vi "SortToneDataForLogging.vi"(7 "Target":T1=enum."4", 10 "element in":cluster{"Enum":T5, "Data":variant}, 11 "TonesLog":T2={"72co"={"Count"=0, "CalVal"=[], "CalLoc"=[], "BeacVal"=[], "BeacLoc"=[], "BeacShift"=[], "Enum"=enum."4", "df"=0.0, "PwrSpectr"=[], "ISpectr"=[], "QSpectr"=[], "Time"=[], "SNR"=[], "AboveThresh"=[], "10Hz_PeakVal"=[], "Phase"=[], "DeltaPhase"=[], "Saturat"={"Meas"=[], "Stage1"=[], "Stage4"=[], "Stage5"=[], "Stage6"=[], "Stage7"=[]}, "10MHz"=FALSE}, "72x"={"Count"=0, "CalVal"=[], "CalLoc"=[], "BeacVal"=[], "BeacLoc"=[], "BeacShift"=[], "Enum"=enum."4", "df"=0.0, "PwrSpectr"=[], "ISpectr"=[], "QSpectr"=[], "Time"=[], "SNR"=[], "AboveThresh"=[], "10Hz_PeakVal"=[], "Phase"=[], "DeltaPhase"=[], "Saturat"={"Meas"=[], "Stage1"=[], "Stage4"=[], "Stage5"=[], "Stage6"=[], "Stage7"=[]}, "10MHz"=FALSE}, "84co"={"Count"=0, "CalVal"=[], "CalLoc"=[], "BeacVal"=[], "BeacLoc"=[], "BeacShift"=[], "Enum"=enum."4", "df"=0.0, "PwrSpectr"=[], "ISpectr"=[], "QSpectr"=[], "Time"=[], "SNR"=[], "AboveThresh"=[], "10Hz_PeakVal"=[], "Phase"=[], "DeltaPhase"=[], "Saturat"={"Meas"=[], "Stage1"=[], "Stage4"=[], "Stage5"=[], "Stage6"=[], "Stage7"=[]}, "10MHz"=FALSE}, "84x"={"Count"=0, "CalVal"=[], "CalLoc"=[], "BeacVal"=[], "BeacLoc"=[], "BeacShift"=[], "Enum"=enum."4", "df"=0.0, "PwrSpectr"=[], "ISpectr"=[], "QSpectr"=[], "Time"=[], "SNR"=[], "AboveThresh"=[], "10Hz_PeakVal"=[], "Phase"=[], "DeltaPhase"=[], "Saturat"={"Meas"=[], "Stage1"=[], "Stage4"=[], "Stage5"=[], "Stage6"=[], "Stage7"=[]}, "10MHz"=FALSE}}) -> (1 "SendToQueue":cluster{"Enum":T5, "Data":variant}, 2 "Full set":bool, 3 "TonesLog w/ New Data":T2={"72co"={"Count"=0, "CalVal"=[], "CalLoc"=[], "BeacVal"=[], "BeacLoc"=[], "BeacShift"=[], "Enum"=enum."4", "df"=0.0, "PwrSpectr"=[], "ISpectr"=[], "QSpectr"=[], "Time"=[], "SNR"=[], "AboveThresh"=[], "10Hz_PeakVal"=[], "Phase"=[], "DeltaPhase"=[], "Saturat"={"Meas"=[], "Stage1"=[], "Stage4"=[], "Stage5"=[], "Stage6"=[], "Stage7"=[]}, "10MHz"=FALSE}, "72x"={"Count"=0, "CalVal"=[], "CalLoc"=[], "BeacVal"=[], "BeacLoc"=[], "BeacShift"=[], "Enum"=enum."4", "df"=0.0, "PwrSpectr"=[], "ISpectr"=[], "QSpectr"=[], "Time"=[], "SNR"=[], "AboveThresh"=[], "10Hz_PeakVal"=[], "Phase"=[], "DeltaPhase"=[], "Saturat"={"Meas"=[], "Stage1"=[], "Stage4"=[], "Stage5"=[], "Stage6"=[], "Stage7"=[]}, "10MHz"=FALSE}, "84co"={"Count"=0, "CalVal"=[], "CalLoc"=[], "BeacVal"=[], "BeacLoc"=[], "BeacShift"=[], "Enum"=enum."4", "df"=0.0, "PwrSpectr"=[], "ISpectr"=[], "QSpectr"=[], "Time"=[], "SNR"=[], "AboveThresh"=[], "10Hz_PeakVal"=[], "Phase"=[], "DeltaPhase"=[], "Saturat"={"Meas"=[], "Stage1"=[], "Stage4"=[], "Stage5"=[], "Stage6"=[], "Stage7"=[]}, "10MHz"=FALSE}, "84x"={"Count"=0, "CalVal"=[], "CalLoc"=[], "BeacVal"=[], "BeacLoc"=[], "BeacShift"=[], "Enum"=enum."4", "df"=0.0, "PwrSpectr"=[], "ISpectr"=[], "QSpectr"=[], "Time"=[], "SNR"=[], "AboveThresh"=[], "10Hz_PeakVal"=[], "Phase"=[], "DeltaPhase"=[], "Saturat"={"Meas"=[], "Stage1"=[], "Stage4"=[], "Stage5"=[], "Stage6"=[], "Stage7"=[]}, "10MHz"=FALSE}}, 4 "Target":T1=enum."4", 5 "10Hz_Time":timestamp, 6 "10Hz_PeakVal":dbl[](array[numeric]))   [LabVIEW 2018]
uses:
  Controls/Enums/LogLoopEnum.ctl
  Controls/Clusts/TonesLogAll.ctl
  Controls/Clusts/ToneLogBuffered.ctl
  Controls/Enums/TargetNumber.ctl
  Controls/Clusts/SaturationMonitorBuffer.ctl
  Controls/Clusts/TargetToneData.ctl
  Controls/Clusts/ChannelToneData.ctl
  Controls/ToneInfoClust.ctl
  Controls/Clusts/SaturationMonitor.ctl
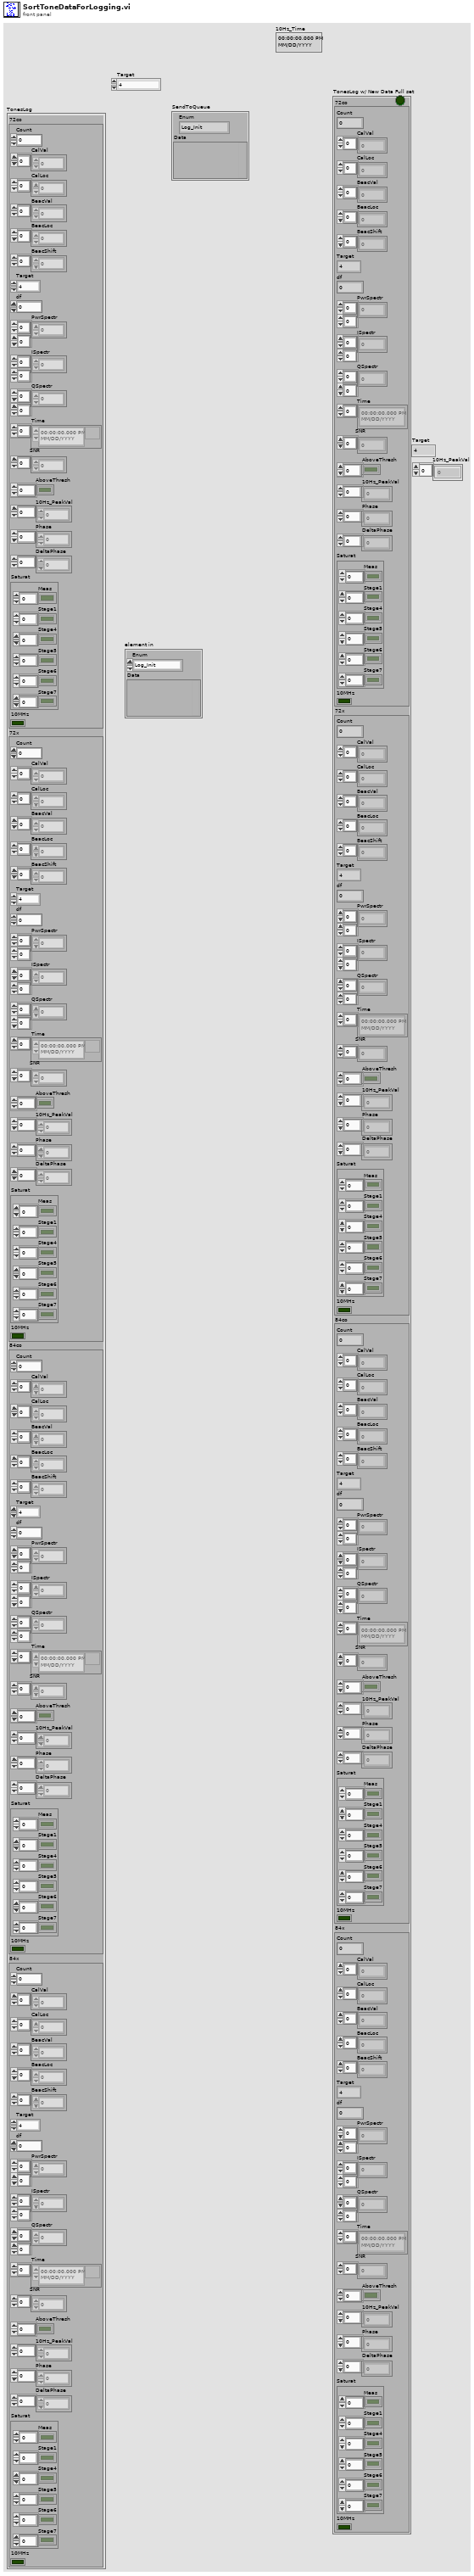
[diagram p1: front panel]
types:
  T1 = typedef "TargetNumber.ctl" = enum16{"1", "2", "3", "4"}
  T2 = typedef "TonesLogAll.ctl" = cluster{"72co":T3, "72x":T3, "84co":T3, "84x":T3}
  T3 = typedef "ToneLogBuffered.ctl" = cluster{"Count":i32, "CalVal":sgl[], "CalLoc":i32[], "BeacVal":sgl[], "BeacLoc":i32[], "BeacShift":i32[], "Enum":T1, "df":dbl, "PwrSpectr":sgl[][], "ISpectr":sgl[][], "QSpectr":sgl[][], "Time":timestamp[], "SNR":sgl[], "AboveThresh":bool[], "10Hz_PeakVal":dbl[], "Phase":sgl[], "DeltaPhase":dbl[], "Saturat":T4, "10MHz":bool}
  T4 = typedef "SaturationMonitorBuffer.ctl" = cluster{"Meas":bool[], "Stage1":bool[], "Stage4":bool[], "Stage5":bool[], "Stage6":bool[], "Stage7":bool[]}
  T5 = typedef "LogLoopEnum.ctl" = enum16{"Log_Init", "Log_Config", "Log_CfgAlarm", "Log_TimeDomain", "Log_Tone", "Log_NoiseTrace", "Log_NoiseSum", "Log_DO", "Log_AI", "Log_TC", "Log_Disdrom", "Log_Weather", "Log_TE", "Log_ADAM", "Log_UPS", "Log_ChkTime", "Log_Alarm", "Log_SSH", "Log_Write", "Log_Exit"}
  T6 = typedef "TargetToneData.ctl" = cluster{"Cal":T7, "Beac":T7, "Time":timestamp[], "Saturat":T9}
  T7 = typedef "ChannelToneData.ctl" = cluster{"Shift_":dbl, "Peak_ToFPGA":dbl, "MaxValue":dbl, "MaxIndex":i32, "Tone":T8, "TimeDomainI":ext[], "TimeDomainQ":ext[], "PwrSpectrum":dbl[], "RunningAvgFreq":dbl, "ISpectPos":dbl[], "ISpectNeg":dbl[], "QSpectPos":dbl[], "QSpectNeg":dbl[], "10Hz_PwrSpectr":dbl[][], "SNR":dbl, "AliasWarn":bool, "10Hz_Peak":dbl[], "ISpect+-":dbl[], "QSpect+-":dbl[], "TimeStamp":timestamp, "I_Index":ext[], "Q_Index":ext[], "10MHz":bool}
  T8 = typedef "ToneInfoClust.ctl" = cluster{"PkLocTrak":dbl, "PkLocDisp":dbl, "df_":dbl, "ZoomPwr":dbl[], "Phase":dbl, "PhaseOld":dbl, "AboveThresh?":bool, "MaxI":dbl, "MaxQ":dbl, "median":dbl, "ISpect":dbl[], "QSpect":dbl[], "DeltaPhase":dbl}
  T9 = typedef "SaturationMonitor.ctl" = cluster{"MeasMean0":dbl, "MeasMean1":dbl, "MeasMax":dbl, "1_Max":dbl, "4_Max":dbl, "5_Max":dbl, "6_Max":dbl, "7_Max":dbl}
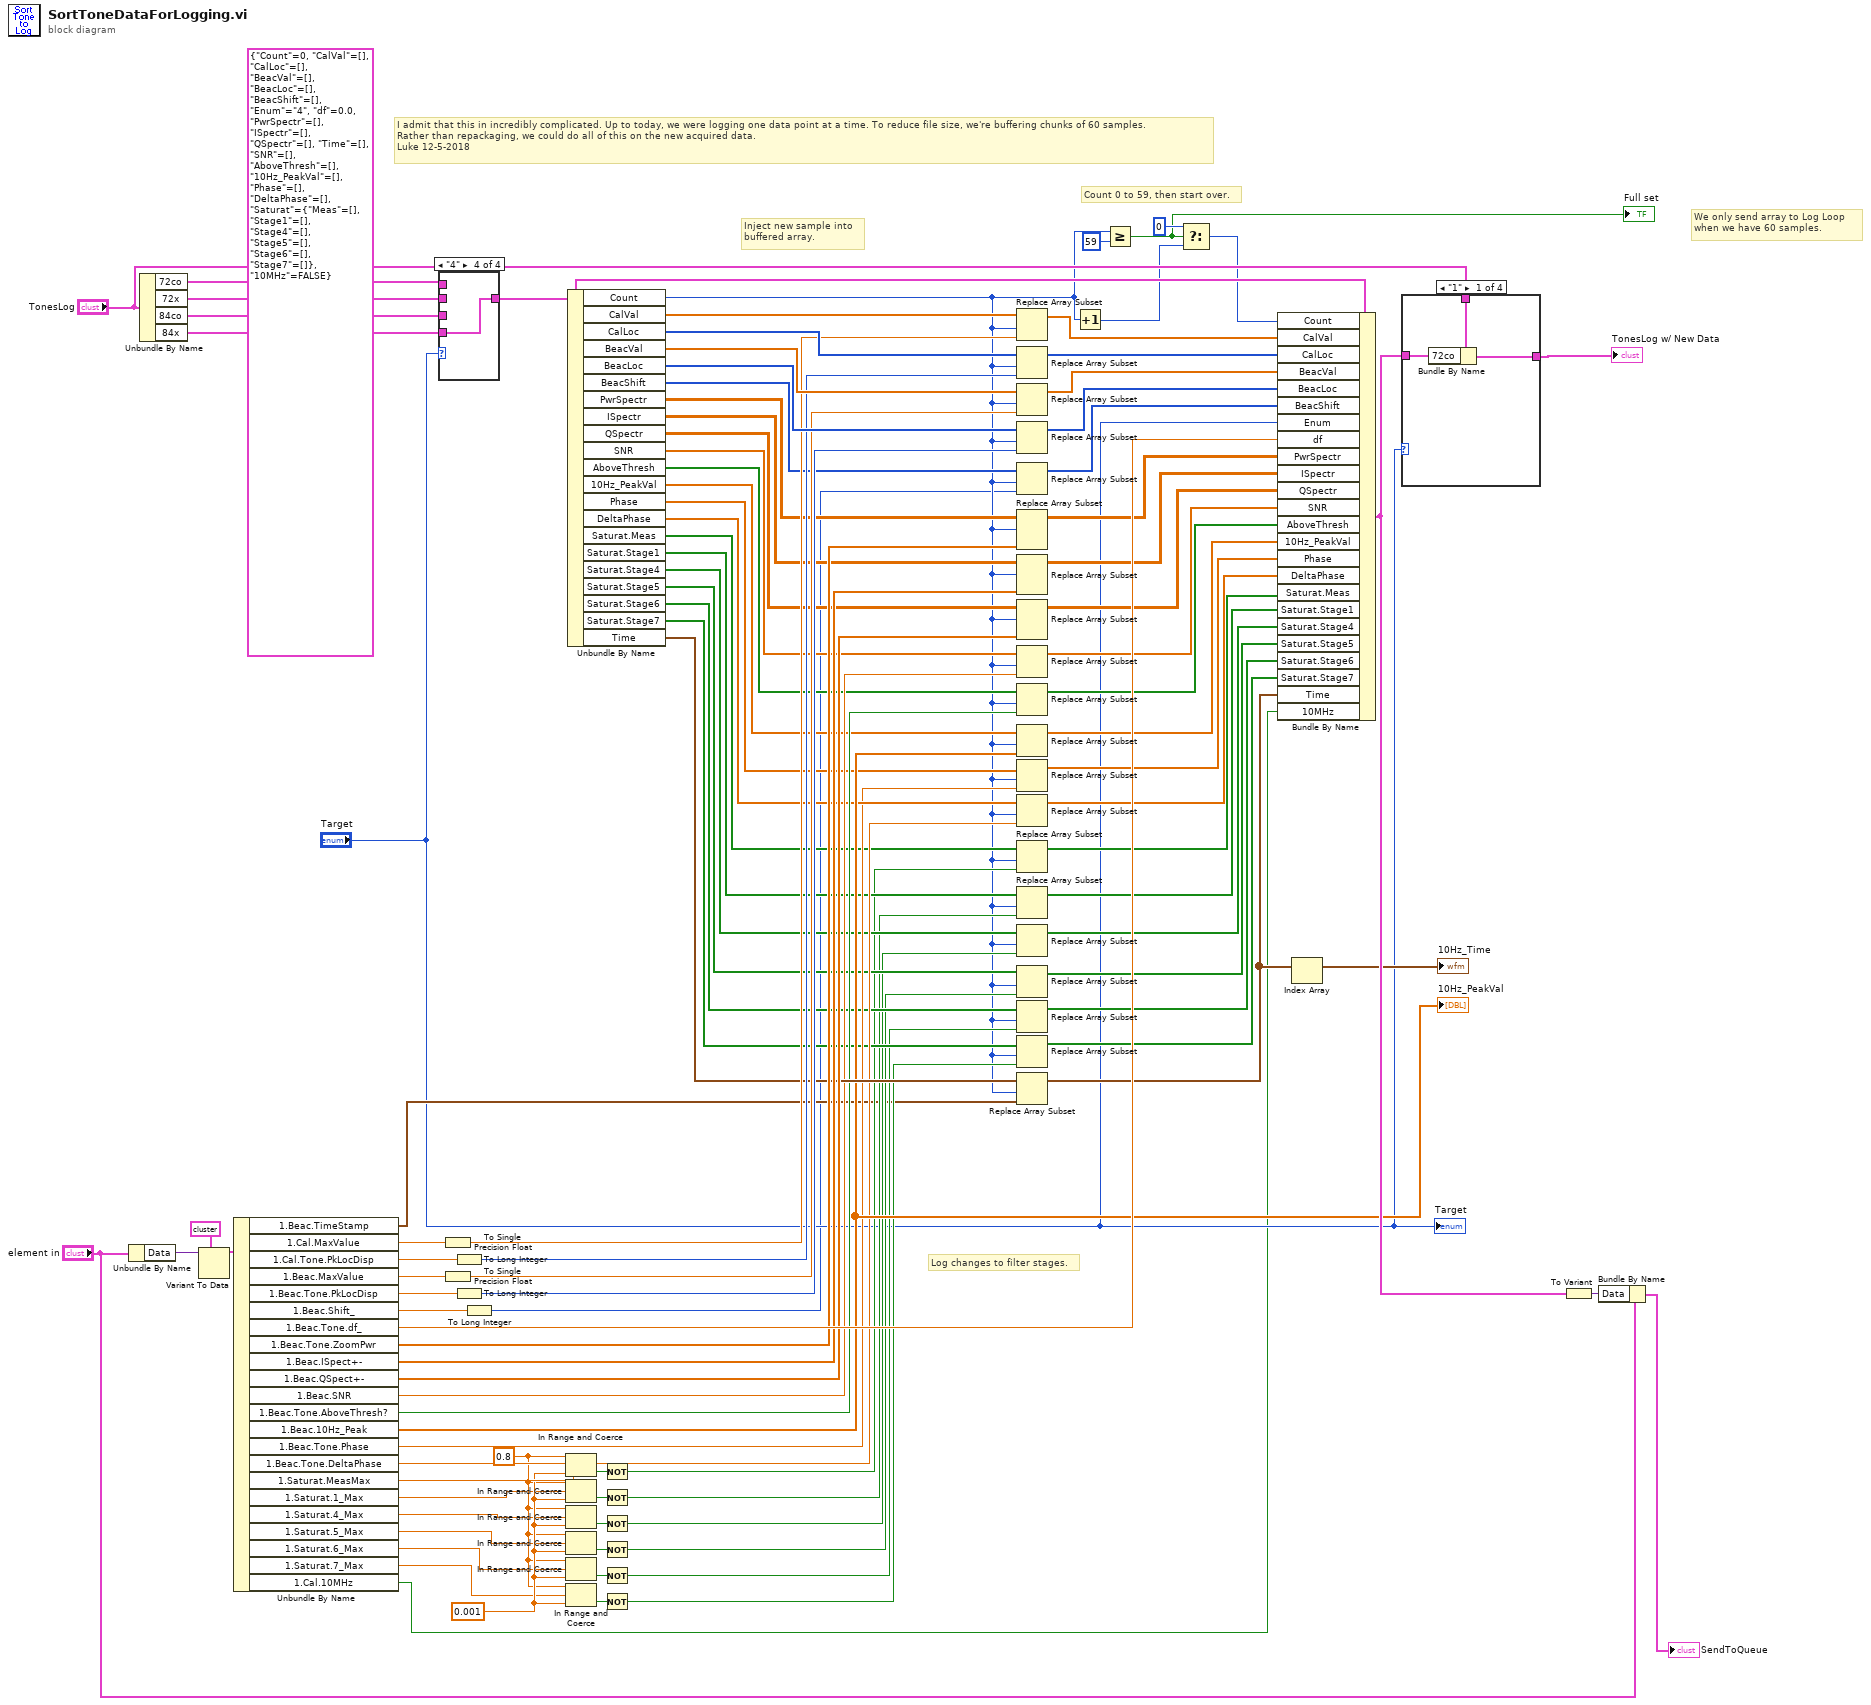
[diagram p0: block diagram]
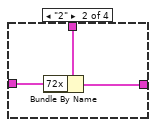
[diagram p2: hidden frame]
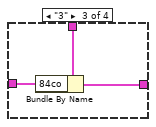
[diagram p3: hidden frame]
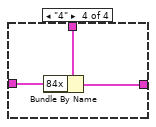
[diagram p4: hidden frame]
diagram:
  (unwired) T3 {"Count"=0, "CalVal"=[], "CalLoc"=[], "BeacVal"=[], "BeacLoc"=[], "BeacShift"=[], "Enum"=enum."4", "df"=0.0, "PwrSpectr"=[], "ISpectr"=[], "QSpectr"=[], "Time"=[], "SNR"=[], "AboveThresh"=[], "10Hz_PeakVal"=[], "Phase"=[], "DeltaPhase"=[], "Saturat"={"Meas"=[], "Stage1"=[], "Stage4"=[], "Stage5"=[], "Stage6"=[], "Stage7"=[]}, "10MHz"=FALSE} ("84x")
  w41 = 0.001 ("upper limit")
  w40 = 0.8 ("upper limit")
  # "Log changes to filter stages."
  # "We only send array to Log Loop\nwhen we have 60 samples."
  # "Inject new sample into\nbuffered array."
  # "Count 0 to 59, then start over."
  # "I admit that this in incredibly complicated. Up to today, we were logging one data point at a time. To reduce file size, we're buffering chunks of 60 samples.\nRather than repackaging, we could do all of this on the new acquired data.\nLuke 12-5-2018"
  n1 = Unbundle By Name("element in") -> ("Data"=w98:variant)
  n2 = Unbundle By Name("TonesLog") -> ("72co"=w102:T3, "72x"=w101:T3, "84co"=w100:T3, "84x"=w99:T3)
  n3 = Variant To Data(type=cluster{"Target":T1, "1":T6} {"Target"=enum."1", "1"={"Cal"={"Shift_"=0.0, "Peak_ToFPGA"=0.0, "MaxValue"=0.0, "MaxIndex"=0, "Tone"={"PkLocTrak"=0.0, "PkLocDisp"=0.0, "df_"=0.0, "ZoomPwr"=[], "Phase"=0.0, "PhaseOld"=0.0, "AboveThresh?"=FALSE, "MaxI"=0.0, "MaxQ"=0.0, "median"=0.0, "ISpect"=[], "QSpect"=[], "DeltaPhase"=0.0}, "TimeDomainI"=[], "TimeDomainQ"=[], "PwrSpectrum"=[], "RunningAvgFreq"=0.0, "ISpectPos"=[], "ISpectNeg"=[], "QSpectPos"=[], "QSpectNeg"=[], "10Hz_PwrSpectr"=[], "SNR"=0.0, "AliasWarn"=FALSE, "10Hz_Peak"=[], "ISpect+-"=[], "QSpect+-"=[], "TimeStamp"=timestamp(0 s since 1904-01-01), "I_Index"=array[12500 elements], "Q_Index"=array[12500 elements], "10MHz"=FALSE}, "Beac"={"Shift_"=0.0, "Peak_ToFPGA"=0.0, "MaxValue"=0.0, "MaxIndex"=0, "Tone"={"PkLocTrak"=0.0, "PkLocDisp"=0.0, "df_"=0.0, "ZoomPwr"=[], "Phase"=0.0, "PhaseOld"=0.0, "AboveThresh?"=FALSE, "MaxI"=0.0, "MaxQ"=0.0, "median"=0.0, "ISpect"=[], "QSpect"=[], "DeltaPhase"=0.0}, "TimeDomainI"=[], "TimeDomainQ"=[], "PwrSpectrum"=[], "RunningAvgFreq"=0.0, "ISpectPos"=[], "ISpectNeg"=[], "QSpectPos"=[], "QSpectNeg"=[], "10Hz_PwrSpectr"=[], "SNR"=0.0, "AliasWarn"=FALSE, "10Hz_Peak"=[], "ISpect+-"=[], "QSpect+-"=[], "TimeStamp"=timestamp(0 s since 1904-01-01), "I_Index"=array[12500 elements], "Q_Index"=array[12500 elements], "10MHz"=FALSE}, "Time"=[], "Saturat"={"MeasMean0"=0.0, "MeasMean1"=0.0, "MeasMax"=0.0, "1_Max"=0.0, "4_Max"=0.0, "5_Max"=0.0, "6_Max"=0.0, "7_Max"=0.0}}} ("Target# and Tone Data"), Variant=w98) -> (data=w97:cluster{"Target":T1, "1":T6})  [unwired: 1 in, 1 out]
  n4 = Unbundle By Name(w97) -> ("1.Beac.TimeStamp"=w5:timestamp, "1.Cal.MaxValue"=w95:dbl, "1.Cal.Tone.PkLocDisp"=w89:dbl, "1.Beac.MaxValue"=w70:dbl, "1.Beac.Tone.PkLocDisp"=w71:dbl, "1.Beac.Shift_"=w7:dbl, "1.Beac.Tone.df_"=w69:dbl, "1.Beac.Tone.ZoomPwr"=w68:dbl[], "1.Beac.ISpect+-"=w67:dbl[], "1.Beac.QSpect+-"=w66:dbl[], "1.Beac.SNR"=w56:dbl, "1.Beac.Tone.AboveThresh?"=w54:bool, "1.Beac.10Hz_Peak"=w49:dbl[], "1.Beac.Tone.Phase"=w44:dbl, "1.Beac.Tone.DeltaPhase"=w43:dbl, "1.Saturat.MeasMax"=w42:dbl, "1.Saturat.1_Max"=w39:dbl, "1.Saturat.4_Max"=w38:dbl, "1.Saturat.5_Max"=w37:dbl, "1.Saturat.6_Max"=w36:dbl, "1.Saturat.7_Max"=w35:dbl, "1.Cal.10MHz"=w2:bool)
  "10Hz_PeakVal" <- w49
  n5 = case shown="\"4\"" "Target" {
    tunnel: w102 -> [w104 _ _ _]
    tunnel: w101 -> [_ w105 _ _]
    tunnel: w100 -> [_ _ w106 _]
    tunnel: w99 -> [_ _ _ w107]
    tunnel: [w104 w105 w106 w107] -> w94
    frame "1", Default {
    }
    frame "2" {
    }
    frame "3" {
    }
    frame "4" {
    }
  }
  n6 = To Single Precision Float(number=w95) -> (single precision float=w75:sgl)
  n7 = To Single Precision Float(number=w70) -> (single precision float=w72:sgl)
  n8 = To Long Integer(number=w89) -> (32bit integer=w74:i32)
  n9 = To Long Integer(number=w71) -> (32bit integer=w73:i32)
  n10 = To Long Integer(number=w7) -> (32bit integer=w1:i32)
  n11 = In Range and Coerce(upper limit=w40, x=w42, lower limit=w41) -> (In Range?=w22:bool)  [unwired: 1 out]
  n12 = In Range and Coerce(upper limit=w40, x=w39, lower limit=w41) -> (In Range?=w20:bool)  [unwired: 1 out]
  n13 = In Range and Coerce(upper limit=w40, x=w38, lower limit=w41) -> (In Range?=w19:bool)  [unwired: 1 out]
  n14 = In Range and Coerce(upper limit=w40, x=w37, lower limit=w41) -> (In Range?=w18:bool)  [unwired: 1 out]
  n15 = In Range and Coerce(upper limit=w40, x=w36, lower limit=w41) -> (In Range?=w17:bool)  [unwired: 1 out]
  n16 = In Range and Coerce(upper limit=w40, x=w35, lower limit=w41) -> (In Range?=w21:bool)  [unwired: 1 out]
  n17 = Unbundle By Name(w94) -> ("Count"=w8:i32, "CalVal"=w96:sgl[], "CalLoc"=w92:i32[], "BeacVal"=w91:sgl[], "BeacLoc"=w90:i32[], "BeacShift"=w10:i32[], "PwrSpectr"=w65:sgl[][], "ISpectr"=w64:sgl[][], "QSpectr"=w63:sgl[][], "SNR"=w57:sgl[], "AboveThresh"=w53:bool[], "10Hz_PeakVal"=w51:dbl[], "Phase"=w48:sgl[], "DeltaPhase"=w46:dbl[], "Saturat.Meas"=w34:bool[], "Saturat.Stage1"=w32:bool[], "Saturat.Stage4"=w30:bool[], "Saturat.Stage5"=w28:bool[], "Saturat.Stage6"=w26:bool[], "Saturat.Stage7"=w24:bool[], "Time"=w59:timestamp[])
  n18 = Not(x=w22) -> (.not. x?=w16:bool)
  n19 = Not(x=w20) -> (.not. x?=w15:bool)
  n20 = Not(x=w19) -> (.not. x?=w14:bool)
  n21 = Not(x=w18) -> (.not. x?=w13:bool)
  n22 = Not(x=w17) -> (.not. x?=w12:bool)
  n23 = Not(x=w21) -> (.not. x?=w11:bool)
  n24 = Replace Array Subset(array=w96, new element=w75, index=w8) -> (w93:sgl[])
  n25 = Replace Array Subset(array=w92, new element=w74, index=w8) -> (w88:i32[])
  n26 = Replace Array Subset(array=w91, new element=w72, index=w8) -> (w87:sgl[])
  n27 = Replace Array Subset(array=w90, new element=w73, index=w8) -> (w86:i32[])
  n28 = Replace Array Subset(array=w10, new element=w1, index=w8) -> (w9:i32[])
  n29 = Replace Array Subset(array=w65, new element=w68, index (row)=w8) -> (w62:sgl[][])  [unwired: 1 in]
  n30 = Replace Array Subset(array=w64, new element=w67, index (row)=w8) -> (w61:sgl[][])  [unwired: 1 in]
  n31 = Replace Array Subset(array=w63, new element=w66, index (row)=w8) -> (w60:sgl[][])  [unwired: 1 in]
  n32 = Replace Array Subset(array=w57, new element=w56, index=w8) -> (w55:sgl[])
  n33 = Replace Array Subset(array=w53, new element=w54, index=w8) -> (w52:bool[])
  n34 = Replace Array Subset(array=w51, new element=w49, index=w8) -> (w50:dbl[])
  n35 = Replace Array Subset(array=w48, new element=w44, index=w8) -> (w47:sgl[])
  n36 = Replace Array Subset(array=w46, new element=w43, index=w8) -> (w45:dbl[])
  n37 = Replace Array Subset(array=w34, new element=w16, index=w8) -> (w33:bool[])
  n38 = Replace Array Subset(array=w32, new element=w15, index=w8) -> (w31:bool[])
  n39 = Replace Array Subset(array=w30, new element=w14, index=w8) -> (w29:bool[])
  n40 = Replace Array Subset(array=w28, new element=w13, index=w8) -> (w27:bool[])
  n41 = Replace Array Subset(array=w26, new element=w12, index=w8) -> (w25:bool[])
  n42 = Replace Array Subset(array=w24, new element=w11, index=w8) -> (w23:bool[])
  n43 = Replace Array Subset(array=w59, new element=w5, index=w8) -> (w6:timestamp[])
  n44 = Increment(x=w8) -> (x+1=w79:i32)
  n45 = Greater Or Equal?(x=w8, y=59) -> (x >= y?=w77:bool)
  "Full set" <- w77
  n46 = Select(t=0, s=w77, f=w79) -> (s? t:f=w78:i32)
  n47 = Bundle By Name(cluster=w94, "Count"=w78, "CalVal"=w93, "CalLoc"=w88, "BeacVal"=w87, "BeacLoc"=w86, "BeacShift"=w9, "Enum"="Target", "df"=w69, "PwrSpectr"=w62, "ISpectr"=w61, "QSpectr"=w60, "SNR"=w55, "AboveThresh"=w52, "10Hz_PeakVal"=w50, "Phase"=w47, "DeltaPhase"=w45, "Saturat.Meas"=w33, "Saturat.Stage1"=w31, "Saturat.Stage4"=w29, "Saturat.Stage5"=w27, "Saturat.Stage6"=w25, "Saturat.Stage7"=w23, "Time"=w6, "10MHz"=w2) -> (w82:T3)
  n48 = Index Array(array=w6) -> (element=→"10Hz_Time":timestamp)  [unwired: 1 in]
  n49 = case shown="\"1\"" "Target" {
    tunnel: "TonesLog" -> [w110 w113 w116 w119]
    tunnel: w82 -> [w109 w112 w115 w118]
    tunnel: [w108 w111 w114 w117] -> w83
    frame "1" {
      n50 = Bundle By Name(cluster=w110, "72co"=w109) -> (w108:T2)
    }
    frame "2" {
      n51 = Bundle By Name(cluster=w113, "72x"=w112) -> (w111:T2)
    }
    frame "3" {
      n52 = Bundle By Name(cluster=w116, "84co"=w115) -> (w114:T2)
    }
    frame "4" {
      n53 = Bundle By Name(cluster=w119, "84x"=w118) -> (w117:T2)
    }
  }
  "TonesLog w/ New Data" <- w83
  n54 = To Variant(anything=w82) -> (Variant=w84:variant)
  n55 = Bundle By Name(cluster="element in", "Data"=w84) -> (→"SendToQueue":cluster{"Enum":T5, "Data":variant})
  "Target" <- "Target"
